vi "SelectTubel.vi"(8 "error in (no error)":errorcluster, 10 "Unique Object Identifier":string, 11 "DataHandler in":refnum<class "DataHandler.lvclass">) -> (0 "error out":errorcluster, 2 "Control Parameter":T1, 3 "DataHandler out":refnum<class "DataHandler.lvclass">)   [LabVIEW 2017, in "DataHandler.lvclass"]
uses:
  DataHandler.lvclass
  DataHandler.lvclass/DataHandler.ctl
  <vilib>/drjdpowell/SQLite Library/SQL Statement/SQL Statement.lvclass/SQL Statement.ctl
  <vilib>/drjdpowell/SQLite Library/SQL Statement/Column I64.vi
  <vilib>/drjdpowell/SQLite Library/SQL Statement/Column DBL.vi
  <vilib>/drjdpowell/SQLite Library/SQL Statement/Step.vi
  <vilib>/drjdpowell/SQLite Library/SQL Statement/Column Type.vi
  <vilib>/drjdpowell/SQLite Library/SQL Statement/Error Message.vi
  <vilib>/drjdpowell/SQLite Library/SQL Statement/Column String.vi
  <vilib>/drjdpowell/SQLite Library/SQL Statement/SQL Statement.lvclass
  <vilib>/drjdpowell/SQLite Library/SQL Connection/Connection.lvclass
panel:
  # "1 - 'Activity (on / off)', \n2 - 'Prioritization', \n3 - 'El. Power Limitation',  \n4 - 'Th. Power Limitation',\n5 - 'Release Time'"
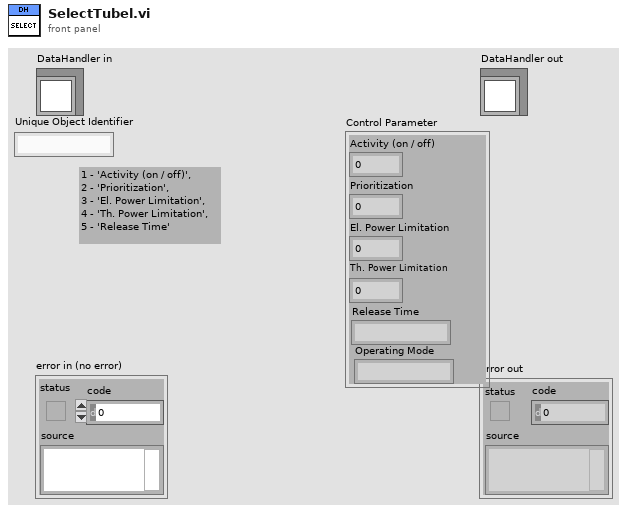
[diagram p1: front panel]
types:
  T1 = cluster{"Activity (on / off)":i64, "Prioritization":i64, "El. Power Limitation":dbl, "Th. Power Limitation":dbl, "Release Time":string, "Operating Mode":string}
  T2 = cluster{"Column:Get Column I64":i64, "Column:Get Column I64":i64, "Column:Get Column DBL":dbl, "Column:Get Column DBL":dbl, "Column:Get Column String":string, "Column:Get Column String":string}
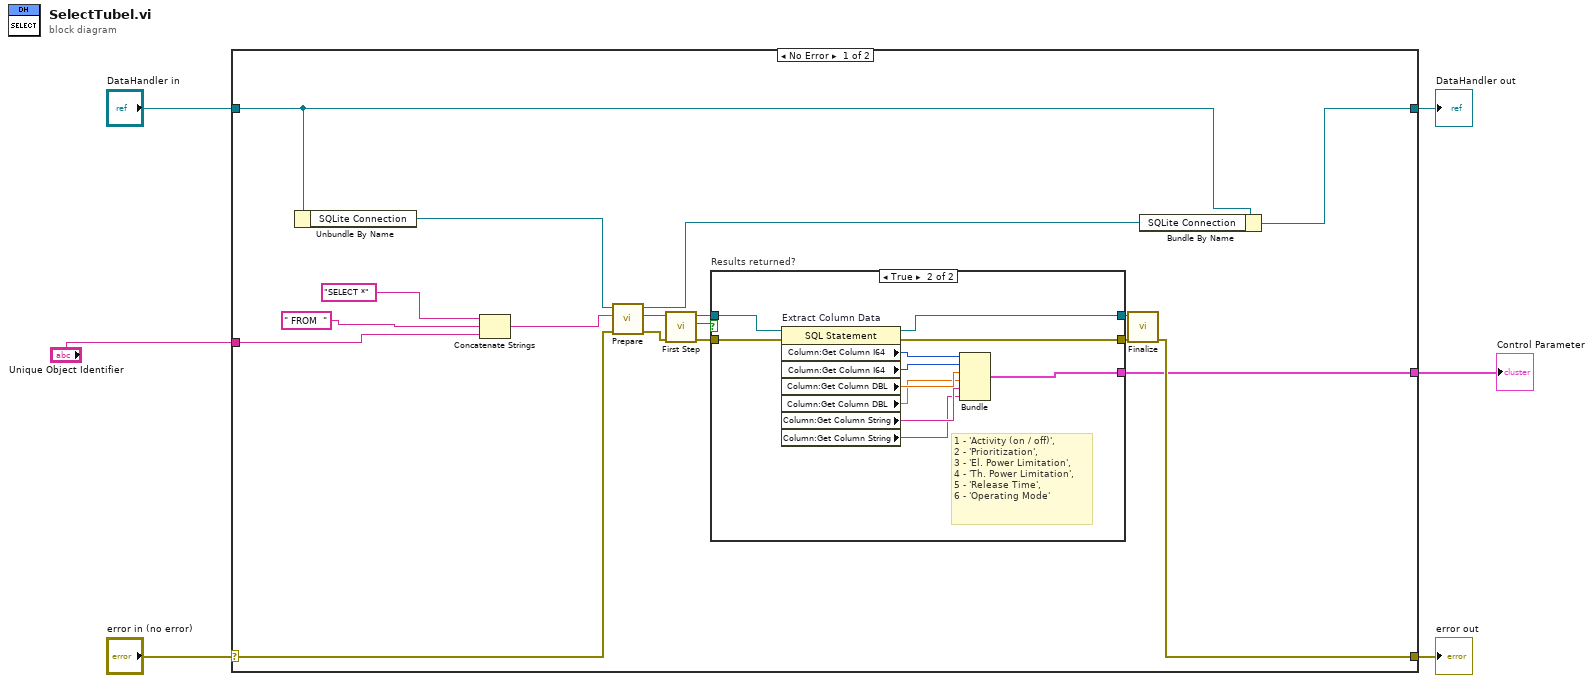
[diagram p0: block diagram]
diagram:
  n1 = case shown="No Error" "error in (no error)" {
    selector: "error in (no error)" -> [w13 w39]
    tunnel: [w12 w39] -> w5
    tunnel: [w15 w38] -> w3
    tunnel: "DataHandler in" -> [w16 w38]
    tunnel: "Unique Object Identifier" -> [w10 _]
    tunnel: [w8 _] -> w1
    frame No Error {
      n2 = Unbundle By Name(w16) -> ("SQLite Connection"=w17:refnum<class "Connection.lvclass">)
      n3 = Concatenate Strings("SELECT *" ("string"), " FROM  " ("string"), w10) -> (w9:string)
      n4 = call <vilib>:"Prepare.vi"("error in (no error)"=w13, "SQL"=w9, "SQLite Connection in"=w17) -> ("error out"=w18:errorcluster, "SQL Statement out"=w19:refnum<class "SQL Statement.lvclass">, "SQLite Connection out"=w14:refnum<class "Connection.lvclass">)  [unwired: 4 in, 2 out]
      n5 = call <vilib>:"First Step.vi"("error in (no error)"=w18, "SQL Statement in"=w19) -> ("error out"=w21:errorcluster, "Row returned"=w20:bool, "SQL Statement out"=w22:refnum<class "SQL Statement.lvclass">)  [unwired: 7 in]
      n6 = case "Results returned?" shown="True" w20 {
        tunnel: [w26 w34] -> w23
        tunnel: [w25 w35] -> w24
        tunnel: w22 -> [w26 w37]
        tunnel: w21 -> [w25 w36]
        tunnel: [_ w28] -> w8
        frame False {
        }
        frame True {
          # "1 - 'Activity (on / off)', \n2 - 'Prioritization', \n3 - 'El. Power Limitation',  \n4 - 'Th. Power Limitation',\n5 - 'Release Time',\n6 - 'Operating Mode'"
          n7 = property on="Extract Column Data" class="SQL Statement"(reference=w37, error in=w36) -> (reference out=w34:refnum<class "SQL Statement.lvclass">, error out=w35:errorcluster, "Column:Get Column I64"=w33:i64, "Column:Get Column I64"=w32:i64, "Column:Get Column DBL"=w31:dbl, "Column:Get Column DBL"=w30:dbl, "Column:Get Column String"=w29:string, "Column:Get Column String"=w27:string)
          n8 = Bundle("Column:Get Column I64"=w33, "Column:Get Column I64"=w32, "Column:Get Column DBL"=w31, "Column:Get Column DBL"=w30, "Column:Get Column String"=w29, "Column:Get Column String"=w27) -> (w28:T2)  [unwired: 1 in]
        }
      }
      n9 = call <vilib>:"Finalize.vi"("error in (no error)"=w24, "SQL Statement in"=w23) -> ("error out"=w12:errorcluster)  [unwired: 9 in]
      n10 = Bundle By Name(cluster=w16, "SQLite Connection"=w14) -> (w15:refnum<class "DataHandler.lvclass">)
    }
    frame Error {
    }
  }
  "error out" <- w5
  "DataHandler out" <- w3
  "Control Parameter" <- w1
